vi "RSNRPZ Set Statistics Scale Ref Level.vi"(8 "error in (no error)":errorcluster, 9 "Reference Level (-30.0 dB)":dbl=-30.0 format="%^.3e", 10 "Channel (1)":i32=1, 11 "VISA session":refnum<visa-resource-name> caption="VISA resource name") -> (0 "error out":errorcluster, 3 "dup VISA session":refnum<visa-resource-name> caption="VISA resource name")   [LabVIEW 2010]
doc: "This VI sets the lower limit of the level range for the analysis result in both Statistics modes. This level can be assigned to the first pixel. The level assigned to the last pixel is equal to the level of the first pixel plus the level range.\n\nRemote-control command(s):\nSENSe:STATistics:SCALE:X:RLEVel"
uses:
  rsnrpz_32.dll
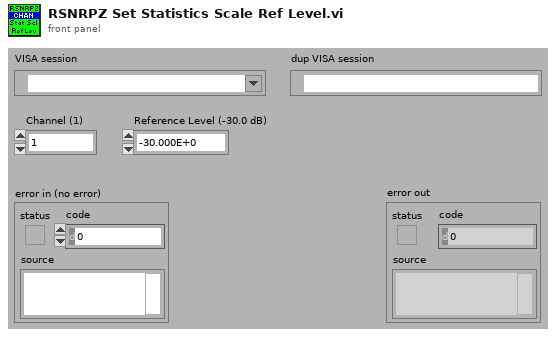
[diagram p1: front panel]
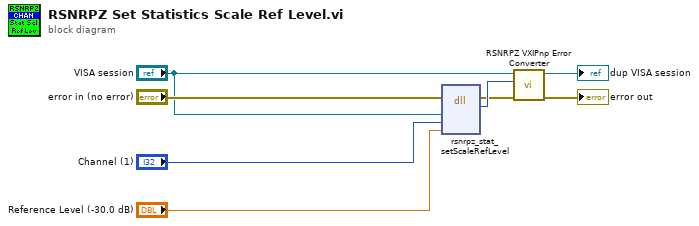
[diagram p0: block diagram]
diagram:
  n1 = dll-call lib="rsnrpz_32.dll" fn="rsnrpz_stat_setScaleRefLevel"(error in="error in (no error)", "Instrument Handle"="VISA session", "Channel"="Channel (1)", "Reference Level"="Reference Level (-30.0 dB)") -> (error out=w5:errorcluster, "Status"=w8:i32)  [unwired: 5 in, 1 out]
  n2 = call <instrlib>:"RSNRPZ VXIPnp Error Converter.vi"("error in"=w5, "VXIPnp error code"=w8, "VISA session"="VISA session") -> ("error out"=→"error out":errorcluster, "dup VISA session"=→"dup VISA session":refnum<visa-resource-name>)  [unwired: 7 in]
